vi "New Element On Board.vi"(7 "New Value Mode":T1, 11 "Board Array":u8[][](array[numeric])) -> (3 "Board Array":u8[][](array[numeric]))   [LabVIEW 2020, in "Game.lvlib"]
uses:
  Game.lvlib
  New Value Mode.ctl
  Element.ctl
  <vilib>/numeric/Random Number (Range) U64.vi
  <vilib>/numeric/sub_Random U32.vi
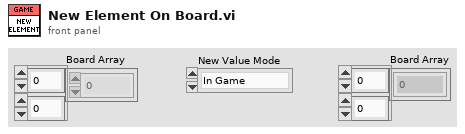
[diagram p1: front panel]
types:
  T1 = typedef "New Value Mode.ctl" = enum16{"In Game", "Initial Game"}
  T2 = enum16{"0", "2", "4", "8", "16", "32", "64", "128", "256", "512", "1024", "2048"}
  T3 = typedef "Element.ctl" = enum16{"0", "2", "4", "8", "16", "32", "64", "128", "256", "512", "1024", "2048"}
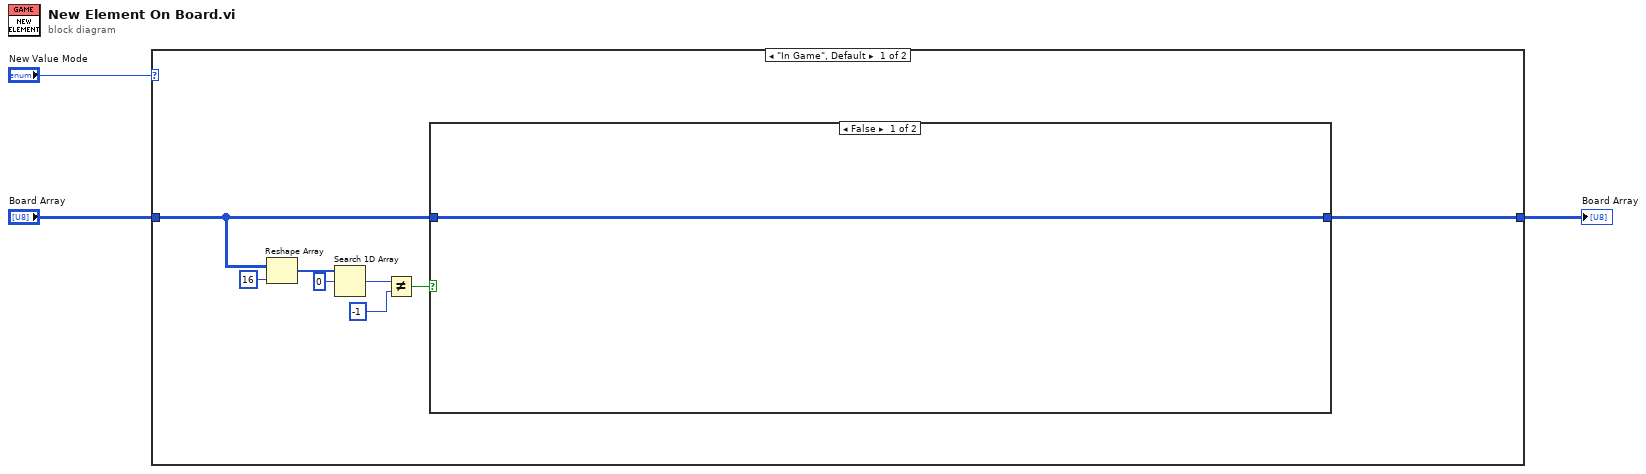
[diagram p0: block diagram]
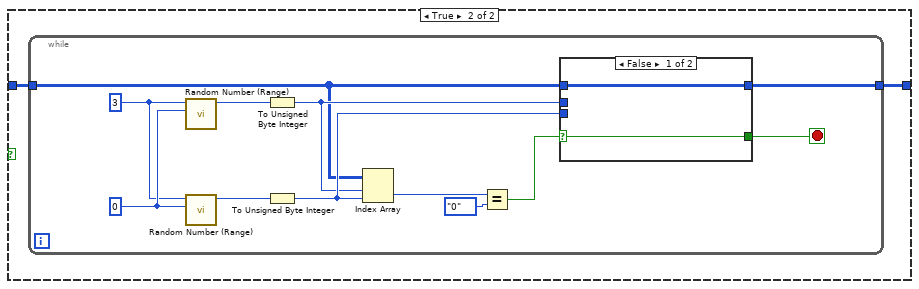
[diagram p2: hidden frame]
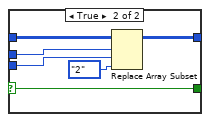
[diagram p3: hidden frame]
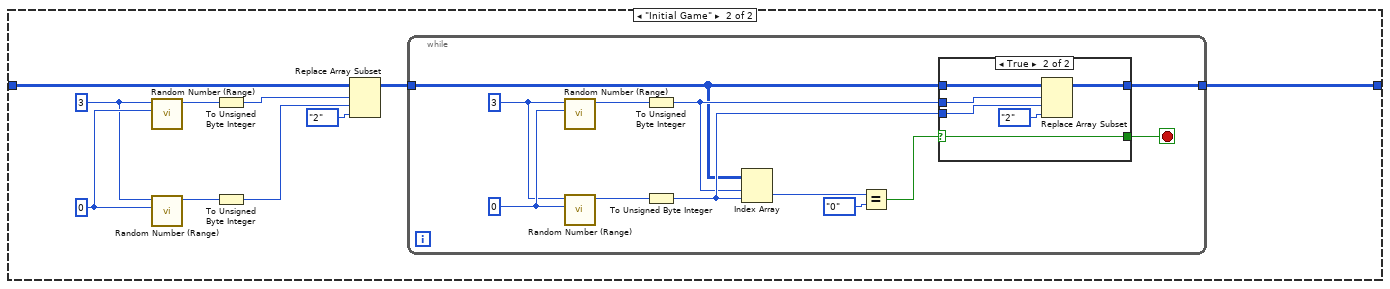
[diagram p4: hidden frame]
diagram:
  n1 = case shown="\"In Game\", Default" "New Value Mode" {
    tunnel: "Board Array" -> [w10 w37]
    tunnel: [w11 w35] -> w1
    frame "In Game", Default {
      n2 = Reshape Array(w10, 16 ("dimension size")) -> (w8:u8[])
      n3 = Search 1D Array(1D array=w8, element=u8 0) -> (index of element=w6:i32)  [unwired: 1 in]
      n4 = Not Equal?(x=w6, y=-1) -> (x != y?=w4:bool)
      n5 = case shown="False" w4 {
        tunnel: [w12 w14] -> w11
        tunnel: w10 -> [w12 w13]
        frame False {
        }
        frame True {
          n6 = while {
            tunnel: w13 -> [w19]
            tunnel: [w16] -> w14
            stop <- w15 stop-if-true
            w25 = u8 3 ("Row")
            w26 = u64 0 ("lower bound (0)")
            n7 = call-poly <vilib>:"Random Number (Range).vi"("lower bound (0)"=w26, "upper bound (100)"=w25) -> ("number"=w17:u64)  [unwired: 9 in]
            n8 = call-poly <vilib>:"Random Number (Range).vi"("lower bound (0)"=w26, "upper bound (100)"=w25) -> ("number"=w18:u64)  [unwired: 9 in]
            n9 = To Unsigned Byte Integer(number=w17) -> (unsigned 8bit integer=w23:u8)
            n10 = To Unsigned Byte Integer(number=w18) -> (unsigned 8bit integer=w24:u8)
            n11 = Index Array(array=w19, index (row)=w23, index (col)=w24) -> (element=w21:u8)
            n12 = Equal?(x=w21, y=T2."0" ("Value")) -> (x = y?=w22:bool)
            n13 = case shown="False" w22 {
              selector: w22 -> [w28 w29]
              tunnel: w19 -> [w27 w34]
              tunnel: w23 -> [_ w32]
              tunnel: w24 -> [_ w31]
              tunnel: [w27 w30] -> w16
              tunnel: [w28 w29] -> w15
              frame False {
              }
              frame True {
                n14 = Replace Array Subset(array=w34, new element=T2."2" ("Value"), index (row)=w32, index (col)=w31) -> (w30:u8[][])
              }
            }
          }
        }
      }
    }
    frame "Initial Game" {
      w43 = u8 3 ("Row")
      w44 = u64 0 ("lower bound (0)")
      n15 = call-poly <vilib>:"Random Number (Range).vi"("lower bound (0)"=w44, "upper bound (100)"=w43) -> ("number"=w41:u64)  [unwired: 9 in]
      n16 = call-poly <vilib>:"Random Number (Range).vi"("lower bound (0)"=w44, "upper bound (100)"=w43) -> ("number"=w42:u64)  [unwired: 9 in]
      n17 = To Unsigned Byte Integer(number=w41) -> (unsigned 8bit integer=w39:u8)
      n18 = To Unsigned Byte Integer(number=w42) -> (unsigned 8bit integer=w38:u8)
      n19 = Replace Array Subset(array=w37, new element=T2."2" ("Value"), index (row)=w39, index (col)=w38) -> (w36:u8[][])
      n20 = while {
        tunnel: w36 -> [w49]
        tunnel: [w46] -> w35
        stop <- w45 stop-if-true
        w55 = u8 3 ("Row")
        w56 = u64 0 ("lower bound (0)")
        n21 = call-poly <vilib>:"Random Number (Range).vi"("lower bound (0)"=w56, "upper bound (100)"=w55) -> ("number"=w47:u64)  [unwired: 9 in]
        n22 = call-poly <vilib>:"Random Number (Range).vi"("lower bound (0)"=w56, "upper bound (100)"=w55) -> ("number"=w48:u64)  [unwired: 9 in]
        n23 = To Unsigned Byte Integer(number=w47) -> (unsigned 8bit integer=w53:u8)
        n24 = To Unsigned Byte Integer(number=w48) -> (unsigned 8bit integer=w54:u8)
        n25 = Index Array(array=w49, index (row)=w53, index (col)=w54) -> (element=w51:u8)
        n26 = Equal?(x=w51, y=Element."0" ("Value")) -> (x = y?=w52:bool)
        n27 = case shown="True" w52 {
          selector: w52 -> [w58 w59]
          tunnel: w49 -> [w57 w64]
          tunnel: w53 -> [_ w62]
          tunnel: w54 -> [_ w61]
          tunnel: [w57 w60] -> w46
          tunnel: [w58 w59] -> w45
          frame False {
          }
          frame True {
            n28 = Replace Array Subset(array=w64, new element=T2."2" ("Value"), index (row)=w62, index (col)=w61) -> (w60:u8[][])
          }
        }
      }
    }
  }
  "Board Array" <- w1
